vi "HGF_Queue.appendData2Variant.vi"(0 "initData":variant, 2 "maxQueueSize (-1)":i32=-1, 5 "error in (no error)":errorcluster) -> (14 "dup initData":variant, 19 "error out":errorcluster)   [LabVIEW 2014, in "HGF_BaseClasses.lvlib" / "HGF_Queue.lvclass"]
doc: "Append initialize data to variant."
uses:
  HGF_Queue.lvclass
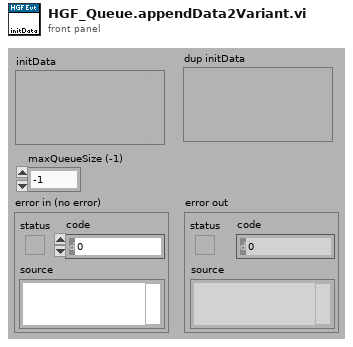
[diagram p1: front panel]
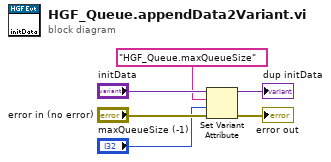
[diagram p0: block diagram]
diagram:
  n1 = Set Variant Attribute(Variant="initData", name="HGF_Queue.maxQueueSize", value="maxQueueSize (-1)", error in="error in (no error)") -> (Variant out=→"dup initData":variant, error out=→"error out":errorcluster)  [unwired: 1 out]
